vi "Disable Default File.vi"(8 "Error In":errorcluster) -> (0 "Error Out":errorcluster)   [LabVIEW 2018, in "Tests.lvlib"]
uses:
  src/Toolkit/Action-Status/Unregister Listener.vi
  src/Toolkit/Support/File/Manager.vi
  src/Toolkit/Support/Manager.vi
  Tests.lvlib
  <vilib>/addons/_JKI Toolkits/Caraya/classes/Test/Test.lvclass
  src/Toolkit/Toolkit.lvlib
  <vilib>/addons/_JKI Toolkits/Caraya/classes/Assert/Assert.lvclass
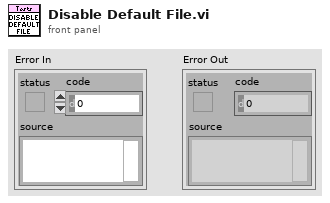
[diagram p1: front panel]
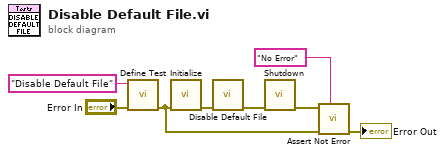
[diagram p0: block diagram]
diagram:
  n1 = call <vilib>:"Define Test.vi"("error in (no error)"="Error In", "Label (VI Title)"="Disable Default File") -> ("error out"=w4:errorcluster)  [unwired: 9 in]
  n2 = call "Initialize.vi"("Error In"=w4) -> ("Error Out"=w7:errorcluster)  [unwired: 10 in]
  n3 = call "Disable Default File.vi"("Error In"=w7) -> ("Error Out"=w1:errorcluster)  [unwired: 10 in]
  n4 = call "Shutdown.vi"("Error In"=w1) -> ("Error Out"=w5:errorcluster)  [unwired: 10 in]
  n5 = call <vilib>:"Assert Not Error.vi"("Label"="No Error", "error in (no error)"=w4, "Not Error?"=w5) -> ("error out"=→"Error Out":errorcluster)  [unwired: 8 in]
